vi "UTF8 LV80.vi"() -> ()   [LabVIEW 2013]
panel:
  out "String":string
  out "text out":string
  in  "text":string
  in  "utf-8 text":string
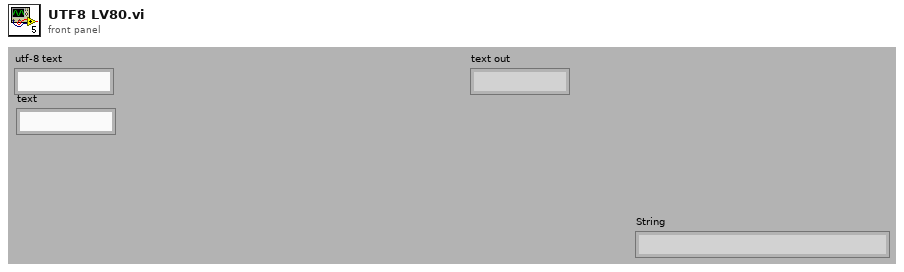
[diagram p1: front panel]
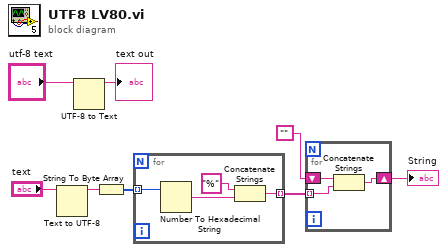
[diagram p0: block diagram]
diagram:
  n1 = Text to UTF-8(11:"text") -> (3:w5:string)  [unwired: 1 in, 1 out]
  n2 = UTF-8 to Text(11:"utf-8 text") -> (3:→"text out":string)  [unwired: 1 in, 1 out]
  n3 = String To Byte Array(string=w5) -> (unsigned byte array=w4:u8[])
  n4 = for {
    tunnel: w4 -> [w12] mode=indexing
    tunnel: [w9] -> w3 mode=indexing
    n5 = Number To Hexadecimal String(2:w12) -> (0:w11:string)  [unwired: 1 in]
    n6 = Concatenate Strings("%" ("string"), w11) -> (w9:string)
  }
  n7 = for {
    tunnel: w3 -> [w13] mode=indexing
    shift-right: [w15] -> w1
    shift-left: "" -> [w14]
    n8 = Concatenate Strings(w14, w13) -> (w15:string)
  }
  "String" <- w1
